vi "Open Device.vi"(8 "error in (no error)":errorcluster, 11 "LightBox in":refnum<class "LightBox.lvclass">) -> (0 "error out":errorcluster, 3 "LightBox out":refnum<class "LightBox.lvclass">)   [LabVIEW 2016, in "LightBox.lvclass"]
uses:
  LightBox.lvclass
  LightBox.lvclass/LightBox.ctl
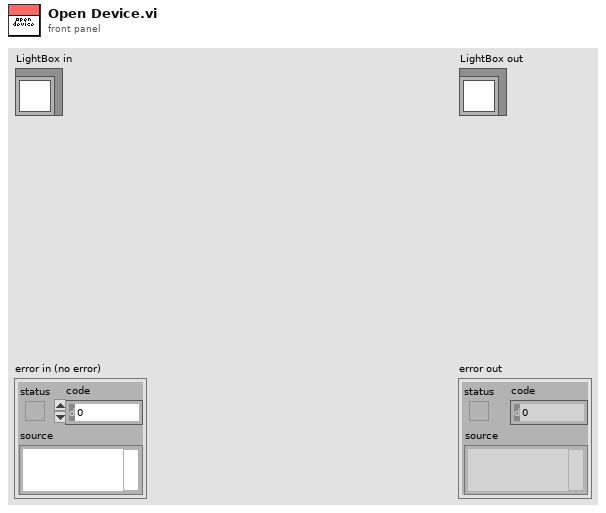
[diagram p1: front panel]
types:
  T1 = typedef "Platinum_MB_SerHandle.ctl" = cluster{"VISAResourceName":string, "Mode":T2, "Timeout":u32, "FlowControl":T3, "Parity":T4, "BaudRate":u32, "SlaveAddress":u8}
  T2 = typedef "Platinum_MB_serMode.ctl" = enum16{"RTU", "ASCII"}
  T3 = typedef "Platinum_MB_serFlowControl.ctl" = enum16{"None", "XON_XOFF", "RTS_CTS", "XON_XOFF_and_RTS_CTS", "DTR_DSR", "XON_XOFF_and_DTR_DSR"}
  T4 = typedef "Platinum_MB_serParity.ctl" = enum16{"None", "Odd", "Even", "Mark", "Space"}
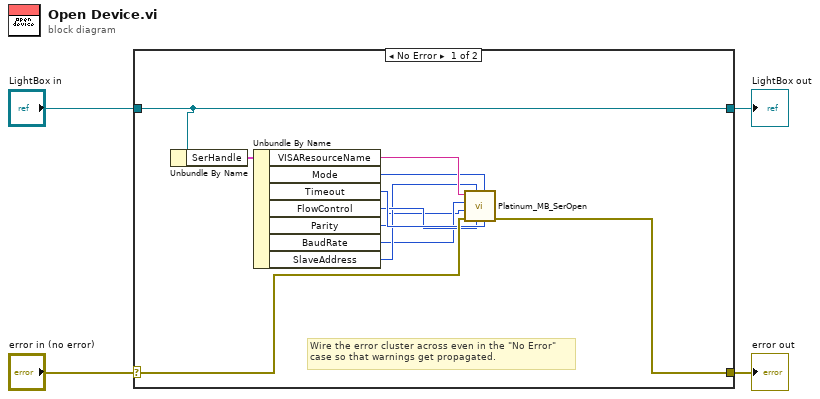
[diagram p0: block diagram]
diagram:
  n1 = case shown="No Error" "error in (no error)" {
    selector: "error in (no error)" -> [w13 w17]
    tunnel: [w12 w17] -> w3
    tunnel: [w15 w16] -> w1
    tunnel: "LightBox in" -> [w15 w16]
    frame No Error {
      # "Wire the error cluster across even in the \"No Error\"\ncase so that warnings get propagated."
      n2 = Unbundle By Name(w15) -> ("SerHandle"=w14:T1)
      n3 = Unbundle By Name(w14) -> ("VISAResourceName"=w11:string, "Mode"=w10:T2, "Timeout"=w9:u32, "FlowControl"=w8:T3, "Parity"=w5:T4, "BaudRate"=w6:u32, "SlaveAddress"=w7:u8)
      n4 = call "Platinum_MB_SerOpen.vi"("Timeout"=w9, "Mode"=w10, "FlowControl"=w8, "SlaveAddress"=w7, "error in"=w13, "Parity"=w5, "BaudRate"=w6, "PortName"=w11) -> ("error out"=w12:errorcluster)  [unwired: 2 in, 1 out]
    }
    frame Error {
    }
  }
  "error out" <- w3
  "LightBox out" <- w1
